vi "GrabToTracker.vi"(0 "IMAQ Refnum":refnum<k11>, 1 "ROI corner pos":cluster{"X":i32, "Y":i32}[](array[cluster]), 5 "Camera In":refnum<queue>, 9 "QTrk Instance":T5, 11 "Camera settings":T1={"Gain [1-4]"=50.0, "Offset"=2, "Mode"=75, "ROIs"=[], "ROI Size"={"X"=0, "Y"=0}, "Number of buffers"=40, "Use hardware multiple-ROI?"=TRUE, "GenericCameraConfig"={"Framerate (Hz)"=60, "Exposure time (us)"=5000, "Image size"={"Width"=1280, "Height"=1024}, "Number of buffers"=30}}, 12 "2D Localization Type (COM)":T4) -> (4 "IMAQ Session Out":refnum<k11>)   [LabVIEW 2011]
uses:
  BeadTracker2.llb/CmdEnum_CameraIn.ctl
  qtrk/QTrk.llb/QTrkZCommandType.ctl
  CameraConfig.ctl
  qtrk/QTrk.llb/QTrkInstance.ctl
  BeadTracker2.llb/Cmd_CameraIn.ctl
  qtrk/QTrk.llb/QTrkLocalizationType.ctl
  BeadTracker2.llb/GenericCameraConfigType.ctl
panel:
  out "Camera settings (out)":T1={"Gain [1-4]"=0.0, "Offset"=0, "Mode"=0, "ROIs"=[], "ROI Size"={"X"=0, "Y"=0}, "Number of buffers"=40, "Use hardware multiple-ROI?"=TRUE, "GenericCameraConfig"={"Framerate (Hz)"=60, "Exposure time (us)"=5000, "Image size"={"Width"=1280, "Height"=1024}, "Number of buffers"=30}}
  out "FPS":i32
  out "Framerate":i32
  out "ROI 4":T3(plugin-control)
  out "result count":i32
  out "ROI 3":T3(plugin-control)
  out "ROI 2":T3(plugin-control)
  out "Frame":i32
  out "Status Information : Lost Frames":u32
  in  "Display mROI image?":bool
  out "ROI 1":T3(plugin-control)
  in  "stop":bool
  out "Actual Width":u32
  # "us"
  # "us"
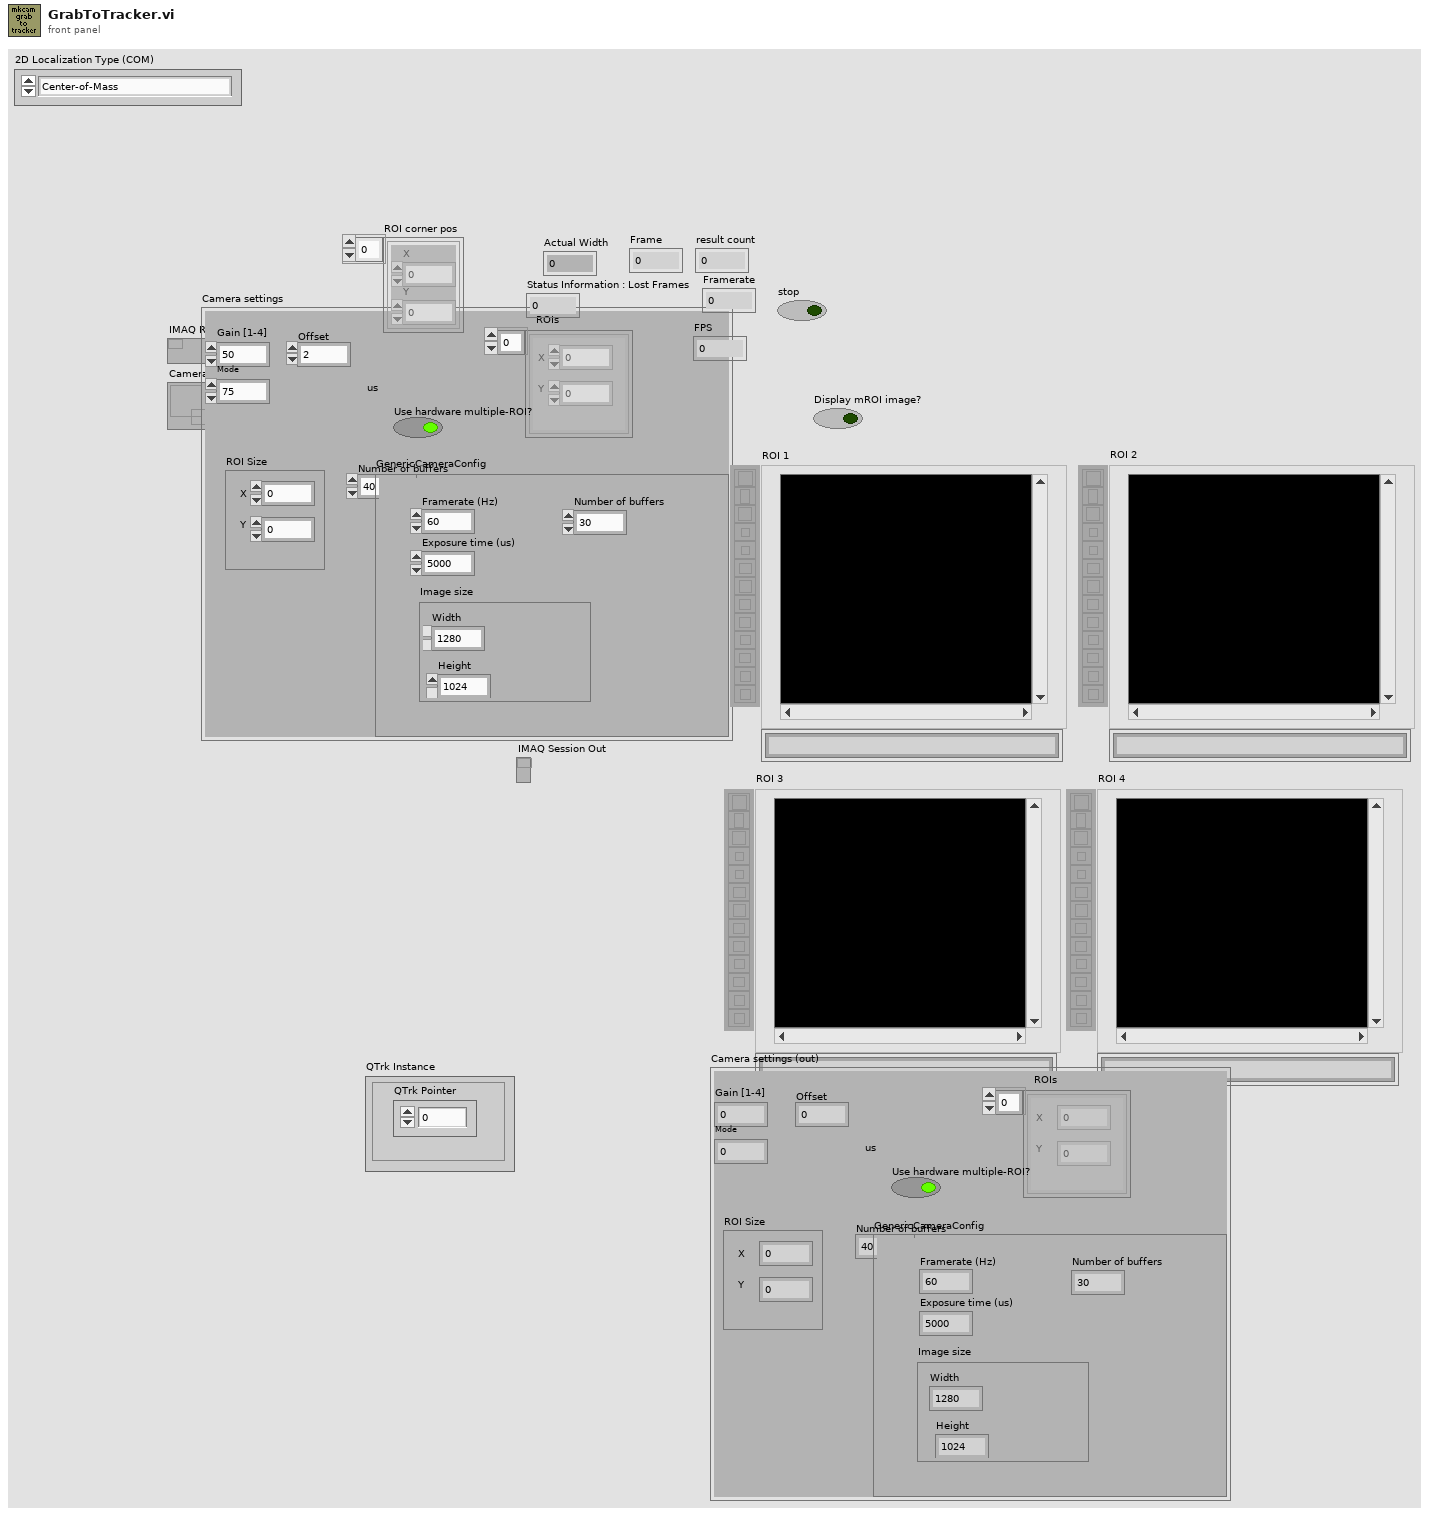
[diagram p1: front panel]
types:
  T1 = typedef "CameraConfig.ctl" = cluster{"Gain [1-4]":sgl, "Offset":i16, "Mode":i16, "ROIs":cluster{"X":i32, "Y":i32}[], "ROI Size":cluster{"X":i32, "Y":i32}, "Number of buffers":i32, "Use hardware multiple-ROI?":bool, "GenericCameraConfig":T2}
  T2 = typedef "GenericCameraConfigType.ctl" = cluster{"Framerate (Hz)":i32, "Exposure time (us)":i32, "Image size":cluster{"Width":i32, "Height":i32}, "Number of buffers":i32}
  T3 = typedef "IMAQ Image.ctl" = refnum<image>
  T4 = typedef "QTrkLocalizationType.ctl" = enum16{"Center-of-Mass", "1D Cross-Correlation", "Quadrant Interpolation", "Gaussian 2D MLE", "QI + ZLUTAlign", "ZLUTAlign"}
  T5 = typedef "QTrkInstance.ctl" = cluster{"QTrk Pointer":u64}
  T6 = typedef "CmdEnum_CameraIn.ctl" = enum32{"Init", "Close", "ShowSettingsDialog", "EndGrab", "GrabZLUT", "GrabToTracker", "GrabToQueue", "AdjustROIs"}
  T7 = typedef "QTrkZCommandType.ctl" = enum16{"Nothing", "ComputeZ", "BuildRadialZLUT", "BuildImageZLUT", "RadialZLUT+ImageZLUT"}
  T8 = typedef "Cmd_CameraIn.ctl" = cluster{"ID":T6, "Msg Data":variant}
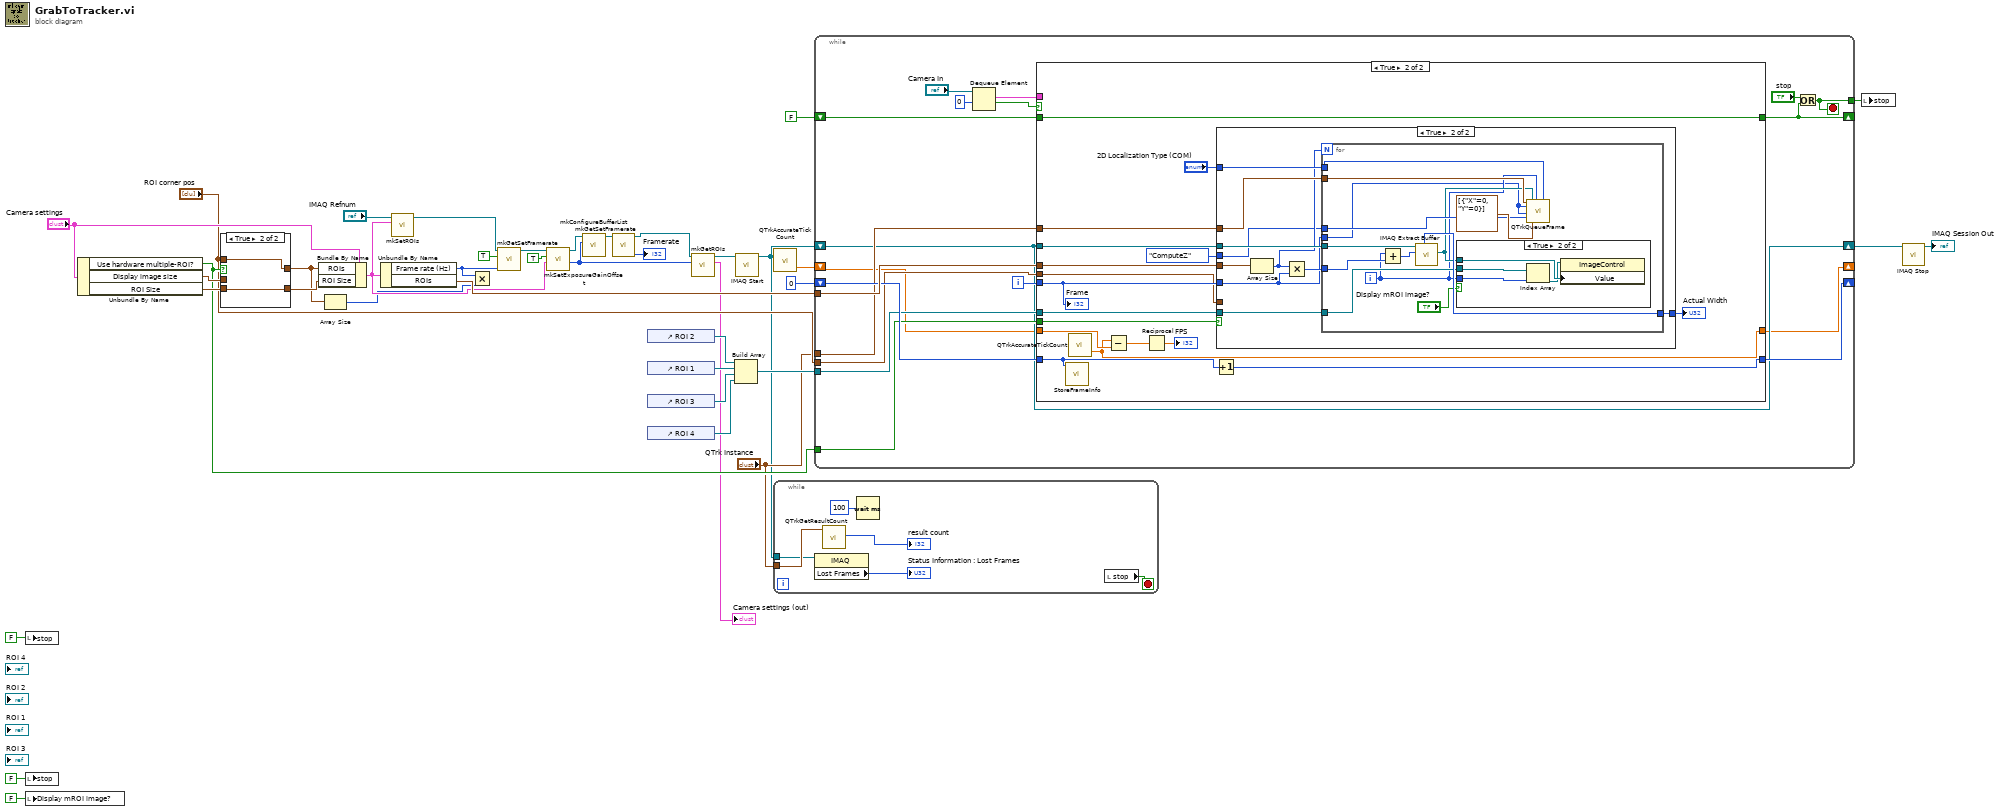
[diagram p0: block diagram]
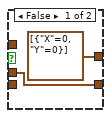
[diagram p2: hidden frame]
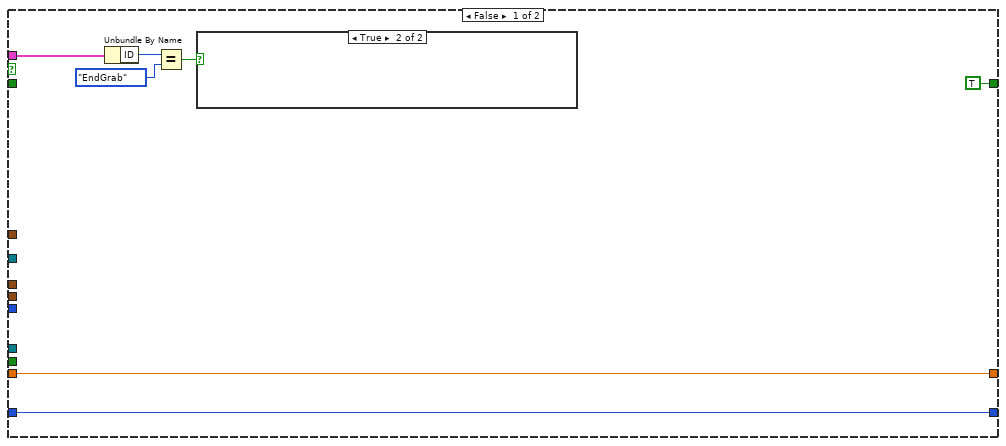
[diagram p3: hidden frame]
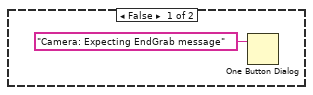
[diagram p4: hidden frame]
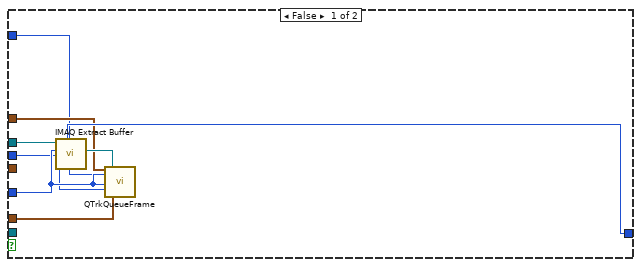
[diagram p5: hidden frame]
diagram:
  n1 = local write "stop"(FALSE ("stop")) -> ()
  n2 = local write "stop"(FALSE ("stop")) -> ()
  n3 = local write "Display mROI image?"(FALSE ("Display mROI image?")) -> ()
  n4 = Unbundle By Name("Camera settings") -> ("Use hardware multiple-ROI?"=w25:bool, "Display image size"=w26:cluster{"X":i32, "Y":i32}, "ROI Size"=w28:cluster{"X":i32, "Y":i32})
  n5 = case shown="True" w25 {
    tunnel: "ROI corner pos" -> [_ w42]
    tunnel: w28 -> [_ w43]
    tunnel: [w40 w43] -> w27
    tunnel: [cluster{"X":i32, "Y":i32}[] [{"X"=0, "Y"=0}] ("f") w42] -> w11
    tunnel: w26 -> [w40 _]
    frame False {
    }
    frame True {
    }
  }
  n6 = Bundle By Name(cluster="Camera settings", "ROIs"=w11, "ROI Size"=w27) -> (w23:T1)
  n7 = Array Size(array=w11) -> (size(s)=w9:i32)
  n8 = Unbundle By Name(w23) -> ("Frame rate (Hz)"=w10:u32, "ROIs"=w34:cluster{"X":i32, "Y":i32}[])
  n9 = call "mkSetROIs.vi"("Camera in"=w23, "IMAQ Refnum in"="IMAQ Refnum") -> ("IMAQ Refnum out"=w5:refnum<k11>)  [unwired: 9 in]
  n10 = Multiply(x=w10, y=w9) -> ()  [unwired: 1 out]
  n11 = call "mkGetSetFramerate.vi"("Framerate"=w10, "Set? (F)"=TRUE, "IMAQ Refnum out"=w5) -> ("IMAQ Refnum (out)"=w37:refnum<k11>)  [unwired: 5 in, 3 out]
  n12 = call "mkSetExposureGainOffset.vi"("Offset"=w23, "Exposure time"=TRUE ("Set? (F)"), "IMAQ Refnum in"=w37) -> ("Offset"=w1:u32, "IMAQ Refnum out"=w32:refnum<k11>)  [unwired: 3 in, 4 out]
  n13 = call "mkConfigureBufferList.vi"("Camera in"=w1, "IMAQ Session"=w32) -> ("IMAQ Session (out)"=w7:refnum<k11>)  [unwired: 9 in]
  n14 = call "mkGetSetFramerate.vi"("IMAQ Refnum out"=w7) -> ("Framerate"=→"Framerate":i32, "IMAQ Refnum (out)"=w4:refnum<k11>)  [unwired: 7 in, 2 out]
  n15 = control-ref of="ROI 2"() -> (w22:refnum<vi>)
  n16 = control-ref of="ROI 1"() -> (w21:refnum<vi>)
  n17 = control-ref of="ROI 3"() -> (w20:refnum<vi>)
  n18 = control-ref of="ROI 4"() -> (w14:refnum<vi>)
  n19 = call "mkGetROIs.vi"("Camera settings"=w1, "IMAQ Refnum in"=w4) -> ("Camera settings (out)"=→"Camera settings (out)":T1, "IMAQ Refnum out"=w3:refnum<k11>)  [unwired: 8 in]
  n20 = Build Array(w22, w21, w20, w14) -> (w19:refnum<vi>[])
  n21 = call <vilib>:"IMAQ Start.vi"("IMAQ Session In"=w3) -> ("IMAQ Session Out"=w15:refnum<k11>)  [unwired: 9 in, 1 out]
  n22 = call "QTrkAccurateTickCount.vi"() -> ("seconds"=w8:dbl)  [unwired: 2 in, 1 out]
  n23 = while {
    tunnel: "QTrk Instance" -> [w48]
    tunnel: w15 -> [w44]
    stop <- w46 stop-if-true
    n24 = property class="IMAQ"(reference=w44) -> ("Lost Frames"=→"Status Information : Lost Frames":u32)  [unwired: 1 in, 2 out]
    n25 = call "QTrkGetResultCount.vi"("QTrk Instance"=w48) -> ("result count"=→"result count":i32)  [unwired: 4 in, 2 out]
    n26 = Wait (ms)(milliseconds to wait=u32 100) -> ()  [unwired: 1 out]
    n27 = local read "stop"() -> (w46:bool)
  }
  n28 = while {
    shift-right: [w53] -> w36
    shift-left: w15 -> [w53]
    shift-right: [w56] -> _
    shift-left: FALSE ("stop") -> [w64]
    tunnel: w34 -> [w63]
    shift-right: [w61] -> _
    shift-left: 0 -> [w62]
    tunnel: w25 -> [w60]
    tunnel: "ROI corner pos" -> [w58]
    tunnel: w19 -> [w55]
    tunnel: "QTrk Instance" -> [w54]
    tunnel: [w52] -> w13
    shift-right: [w50] -> _
    shift-left: w8 -> [w51]
    i -> [w65]
    stop <- w52 stop-if-true
    n29 = Dequeue Element(queue="Camera In", timeout in ms (-1)=0) -> (element=w66:T8, timed out?=w68:bool)  [unwired: 1 in, 2 out]
    n30 = case shown="True" w68 {
      tunnel: w66 -> [w75 _]
      tunnel: w65 -> [_ w93]
      tunnel: w53 -> [_ w83]
      tunnel: [TRUE ("stop") w92] -> w56
      tunnel: w64 -> [_ w92]
      tunnel: w63 -> [_ w91]
      tunnel: w54 -> [_ w81]
      tunnel: w62 -> [w70 w90]
      tunnel: [w70 w89] -> w61
      tunnel: w60 -> [_ w88]
      tunnel: w58 -> [_ w85]
      tunnel: w55 -> [_ w82]
      tunnel: w51 -> [w69 w80]
      tunnel: [w69 w79] -> w50
      frame False {
        n31 = Unbundle By Name(w75) -> ("ID"=w74:T6)
        n32 = Equal?(x=w74, y=CmdEnum_CameraIn."EndGrab") -> (x = y?=w72:bool)
        n33 = case shown="True" w72 {
          frame False {
            n34 = One Button Dialog(message="Camera: Expecting EndGrab message") -> ()  [unwired: 1 in, 1 out]
          }
          frame True {
          }
        }
      }
      frame True {
        n35 = call "StoreFrameInfo.vi"("Timestamp"=w90) -> ()  [unwired: 11 in]
        n36 = call "QTrkAccurateTickCount.vi"() -> ("seconds"=w79:dbl)  [unwired: 2 in, 1 out]
        n37 = Subtract(x=w79, y=w80) -> (x-y=w78:dbl)
        n38 = Reciprocal(x=w78) -> (1/x=→"FPS":dbl)
        n39 = Increment(x=w90) -> (x+1=w89:i32)
        n40 = case shown="True" w88 {
          tunnel: w93 -> [w96 w102]
          tunnel: w83 -> [w101 w111]
          tunnel: w91 -> [_ w107]
          tunnel: w81 -> [w98 w110]
          tunnel: [w100 w109] -> w87
          tunnel: "2D Localization Type (COM)" -> [w95 w108]
          tunnel: w85 -> [w97 _]
          tunnel: QTrkZCommandType."ComputeZ" ("Z Command (None)") -> [w94 w104]
          tunnel: w82 -> [_ w103]
          frame False {
            n41 = call <vilib>:"IMAQ Extract Buffer.vi"("Buffer to extract"=w96, "IMAQ Session In"=w101) -> ("Image Out"=w99:T3, "Actual Width"=w100:u32)  [unwired: 4 in, 4 out]
            n42 = call "QTrkQueueFrame.vi"("QTrk Instance"=w98, "frame#"=w96, "timestamp"=w96, 4:w94, "Image"=w99, "ROI Positions (corner-based)"=w97, 12:w95) -> ()  [unwired: 10 in, 3 out]
          }
          frame True {
            n43 = Array Size(array=w107) -> (size(s)=w106:i32)
            n44 = Multiply(x=w106, y=w102) -> (x*y=w105:i32)
            n45 = for {
              N: w106 -> [_]
              tunnel: w111 -> [w124]
              tunnel: w110 -> [w123]
              tunnel: w108 -> [w122]
              tunnel: [w121] -> w109
              tunnel: w105 -> [w120]
              tunnel: w104 -> [w118]
              tunnel: w103 -> [w115]
              tunnel: w102 -> [w113]
              i -> [w114]
              n46 = Add(x=w114, y=w120) -> (x+y=w112:i32)
              n47 = call <vilib>:"IMAQ Extract Buffer.vi"("Buffer to extract"=w112, "IMAQ Session In"=w124) -> ("Image Out"=w116:T3, "Actual Width"=w121:u32)  [unwired: 4 in, 4 out]
              n48 = case shown="True" "Display mROI image?" {
                tunnel: w116 -> [_ w126]
                tunnel: w115 -> [_ w128]
                tunnel: w114 -> [_ w127]
                frame False {
                }
                frame True {
                  n49 = Index Array(array=w128, index=w127) -> (element=w125:refnum<vi>)
                  n50 = property on="Property Node" class="ImageControl"(reference=w125, "Value"=w126) -> ()  [unwired: 1 in, 2 out]
                }
              }
              n51 = call "QTrkQueueFrame.vi"("QTrk Instance"=w123, "frame#"=w113, "timestamp"=w113, 4:w118, "Image"=w116, "ROI Positions (corner-based)"=cluster{"X":i32, "Y":i32}[] [{"X"=0, "Y"=0}], "ZLUT Index offset (0)"=w114, 12:w122) -> ()  [unwired: 9 in, 3 out]
            }
          }
        }
        "Actual Width" <- w87
        "Frame" <- w93
      }
    }
    n52 = Or(x="stop", y=w56) -> (x .or. y?=w52:bool)
  }
  n53 = local write "stop"(w13) -> ()
  n54 = call <vilib>:"IMAQ Stop.vi"("IMAQ Session In"=w36) -> ("IMAQ Session Out"=→"IMAQ Session Out":refnum<k11>)  [unwired: 9 in, 1 out]
